vi "Trajectory_SampleReverseTEST_ORIENT.vi"(9 "Time":dbl, 11 "InputTRAJECTORY":T5 {"States"."POSE"."ROTATION"."SIN" format="%13.4f"; "States"."POSE"."ROTATION"."COS" format="%13.4f"; "States"."POSE"."ROTATION"."VALUE" format="%13.4f"; "States"."POSE"."TRANSLATION"."Y" format="%14.3f"; "States"."POSE"."TRANSLATION"."X" format="%14.3f"; "TotalTImeSecs" format="%20.3f"}) -> (3 "OutputTRAJ_STATE":T1={"TimeSeconds"=0.0, "Velocity"=0.0, "Acceleration"=0.0, "POSE"={"TRANSLATION"={"X"=0.0, "Y"=0.0}, "ROTATION"={"VALUE"=0.0, "COS"=1.0, "SIN"=0.0}}, "Curvature"=0.0} {"POSE"."ROTATION"."SIN" format="%13.4f"; "POSE"."ROTATION"."COS" format="%13.4f"; "POSE"."ROTATION"."VALUE" format="%13.4f"; "POSE"."TRANSLATION"."Y" format="%14.3f"; "POSE"."TRANSLATION"."X" format="%14.3f"})   [LabVIEW 2019]
doc: "Sample the trajectory at a point in time. The trajectory is sampled in reverse such that the ending time becomes 0 and the beginning time is the maximum time. The selected trajectory state is then transformed to be relative to end of the trajectory.\n\nThis routine does not exist in WPILIB\n \nParameters:\n - InputTrajectory - The Trajectory data structure\n - time - The point in time since the beginning of the trajectory to sample. (seconds)\n\nReturns:\n - OutputTrajState - The state at that point in time."
uses:
  <vilib>/Rock Robotics/WPI/ThirdParty/JAS_Junk/TrajLib/TRAJECTORY.ctl
  <vilib>/Rock Robotics/WPI/ThirdParty/JAS_Junk/TrajLib/TRAJ_STATE.ctl
  <vilib>/Rock Robotics/WPI/ThirdParty/JAS_Junk/TrajLib/POSE2D.ctl
  <vilib>/Rock Robotics/WPI/ThirdParty/JAS_Junk/TrajLib/TRANSLATION2D.ctl
  <vilib>/Rock Robotics/WPI/ThirdParty/JAS_Junk/TrajLib/ROTATION2D.ctl
  <vilib>/Rock Robotics/WPI/ThirdParty/JAS_Junk/TrajLib/Rotation_CreateAngle.vi
  <vilib>/Rock Robotics/WPI/ThirdParty/JAS_Junk/TrajLib/Translation_Create.vi
  <vilib>/Rock Robotics/WPI/ThirdParty/JAS_Junk/TrajLib/Rotation_UnaryMinus.vi
  <vilib>/Rock Robotics/WPI/ThirdParty/JAS_Junk/TrajLib/Translation_RotateBy.vi
  <vilib>/Rock Robotics/WPI/ThirdParty/JAS_Junk/TrajLib/Translation_Minus.vi
  <vilib>/Rock Robotics/WPI/ThirdParty/JAS_Junk/TrajLib/Rotation_Minus.vi
  <vilib>/Rock Robotics/WPI/ThirdParty/JAS_Junk/TrajLib/Translation_Plus.vi
  <vilib>/Rock Robotics/WPI/ThirdParty/JAS_Junk/TrajLib/Rotation_Plus.vi
  <vilib>/Rock Robotics/WPI/ThirdParty/JAS_Junk/TrajLib/Pose_New_TRRO.vi
  <vilib>/Rock Robotics/WPI/ThirdParty/JAS_Junk/TrajLib/Rotation_RotateBy.vi
  <vilib>/Rock Robotics/WPI/ThirdParty/JAS_Junk/TrajLib/Rotation_CreateXY.vi
  <vilib>/Rock Robotics/WPI/ThirdParty/JAS_Junk/TrajLib/Util_CalcDist.vi
  <vilib>/Rock Robotics/WPI/ThirdParty/JAS_Junk/TrajLib/Trajectory_Library.lvlib
panel:
  # "NOTE  ----\nTHIS IS A WORK\nIN PROGRESS.\nIT ISN'T DONE AND\nDOES NOT WORK\nCORRECTLY!"
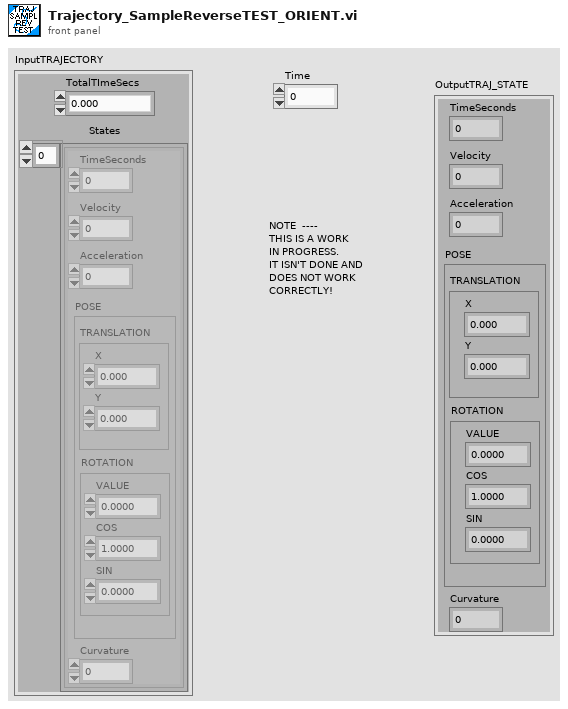
[diagram p1: front panel]
types:
  T1 = typedef "Trajectory_Library.lvlib/TRAJ_STATE.ctl" = cluster{"TimeSeconds":dbl, "Velocity":dbl, "Acceleration":dbl, "POSE":T2, "Curvature":dbl}
  T2 = typedef "Trajectory_Library.lvlib/POSE2D.ctl" = cluster{"TRANSLATION":T3, "ROTATION":T4}
  T3 = typedef "Trajectory_Library.lvlib/TRANSLATION2D.ctl" = cluster{"X":dbl, "Y":dbl}
  T4 = typedef "Trajectory_Library.lvlib/ROTATION2D.ctl" = cluster{"VALUE":dbl, "COS":dbl, "SIN":dbl}
  T5 = typedef "Trajectory_Library.lvlib/TRAJECTORY.ctl" = cluster{"TotalTImeSecs":dbl, "States":T1[]}
  T6 = typedef "Trajectory_Library.lvlib/TRANSFORM2D.ctl" = cluster{"TRANSLATION":T3, "ROTATION":T4}
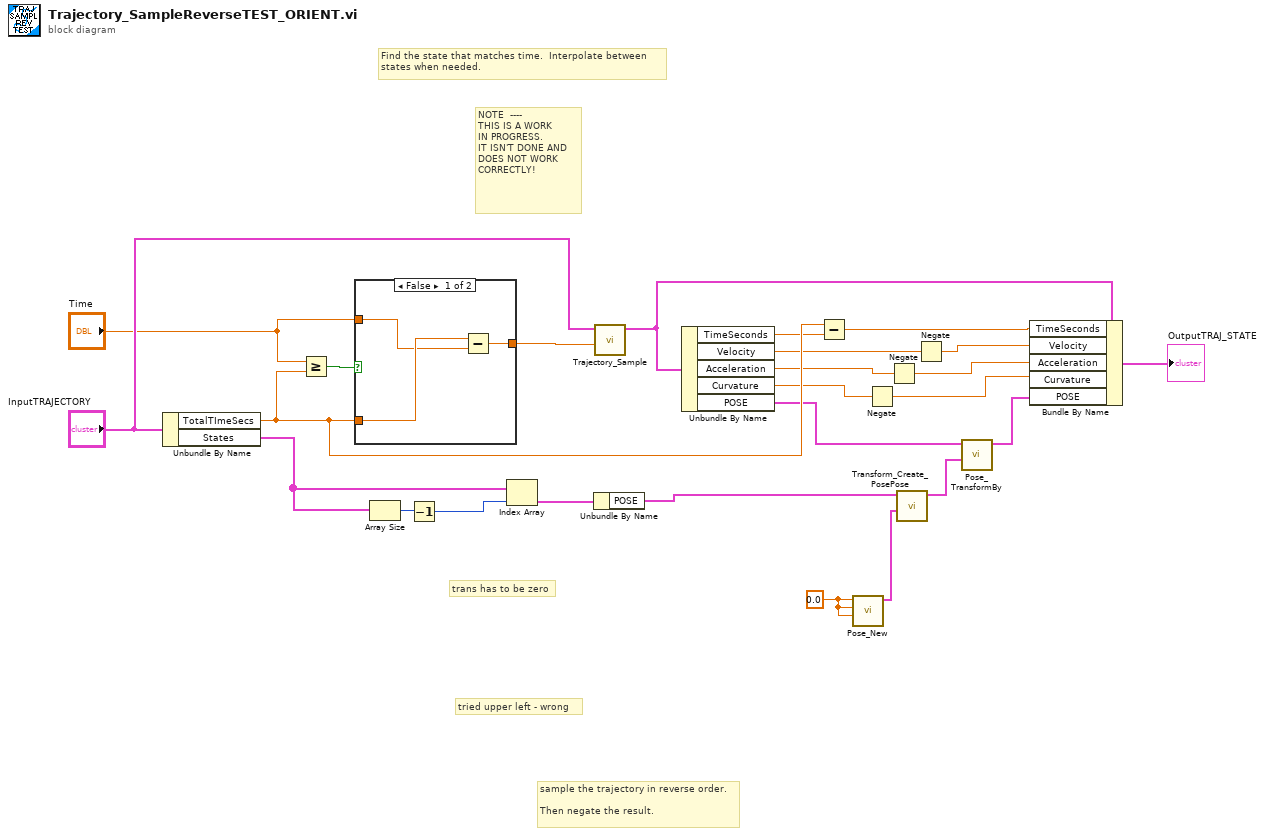
[diagram p0: block diagram]
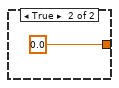
[diagram p2: hidden frame]
diagram:
  w2 = 0.0 ("X")
  # "NOTE  ----\nTHIS IS A WORK\nIN PROGRESS.\nIT ISN'T DONE AND\nDOES NOT WORK\nCORRECTLY!"
  # "tried upper left - wrong"
  # "trans has to be zero"
  # "sample the trajectory in reverse order.\n\nThen negate the result."
  # "Find the state that matches time.  Interpolate between\nstates when needed."
  n1 = Unbundle By Name("InputTRAJECTORY") -> ("TotalTImeSecs"=w19:dbl, "States"=w21:T1[])
  n2 = Greater Or Equal?(x="Time", y=w19) -> (x >= y?=w25:bool)
  n3 = case shown="False" w25 {
    tunnel: [w26 0.0] -> w7
    tunnel: w19 -> [w28 _]
    tunnel: "Time" -> [w27 _]
    frame False {
      n4 = Subtract(x=w28, y=w27) -> (x-y=w26:dbl)
    }
    frame True {
    }
  }
  n5 = Array Size(array=w21) -> (size(s)=w23:i32)
  n6 = Decrement(x=w23) -> (x-1=w22:i32)
  n7 = Index Array(array=w21, index=w22) -> (element=w10:T1)
  n8 = Unbundle By Name(w10) -> ("POSE"=w3:T2)
  n9 = call <vilib>:"Trajectory_Sample.vi"("Time"=w7, "InputTRAJECTORY"="InputTRAJECTORY") -> ("OutputTRAJ_STATE"=w20:T1)  [unwired: 9 in]
  n10 = Unbundle By Name(w20) -> ("TimeSeconds"=w18:dbl, "Velocity"=w16:dbl, "Acceleration"=w14:dbl, "Curvature"=w13:dbl, "POSE"=w5:T2)
  n11 = Subtract(x=w19, y=w18) -> (x-y=w17:dbl)
  n12 = call <vilib>:"Pose_New.vi"("Heading"=w2, "Y"=w2, "X"=w2) -> ("out POSe"=w1:T2)  [unwired: 8 in]
  n13 = Negate(x=w13) -> (-x=w11:dbl)
  n14 = Negate(x=w14) -> (-x=w12:dbl)
  n15 = call <vilib>:"Transform_Create_PosePose.vi"("last POSE"=w1, "initial POSE"=w3) -> ("TRANSFORM"=w9:T6)  [unwired: 9 in]
  n16 = Negate(x=w16) -> (-x=w15:dbl)
  n17 = call <vilib>:"Pose_TransformBy.vi"("other TRANSFORM"=w9, "in POSE"=w5) -> ("out POSE"=w4:T2)  [unwired: 9 in]
  n18 = Bundle By Name(cluster=w20, "TimeSeconds"=w17, "Velocity"=w15, "Acceleration"=w12, "Curvature"=w11, "POSE"=w4) -> (→"OutputTRAJ_STATE":T1)
